vi "Send Email Notification.vi"(5 "Send Email Notification":bool, 7 "Email Notification Cluster (in)":T1, 8 "Error IN":errorcluster, 9 "message":string, 10 "Email Subject":string="[No Subject]", 11 "recipients":string[](array[string])) -> (0 "error out":errorcluster)   [LabVIEW 2012]
uses:
  Controls/Ping address and email notify.ctl
  NewNI_SMTPEmail.lvlib
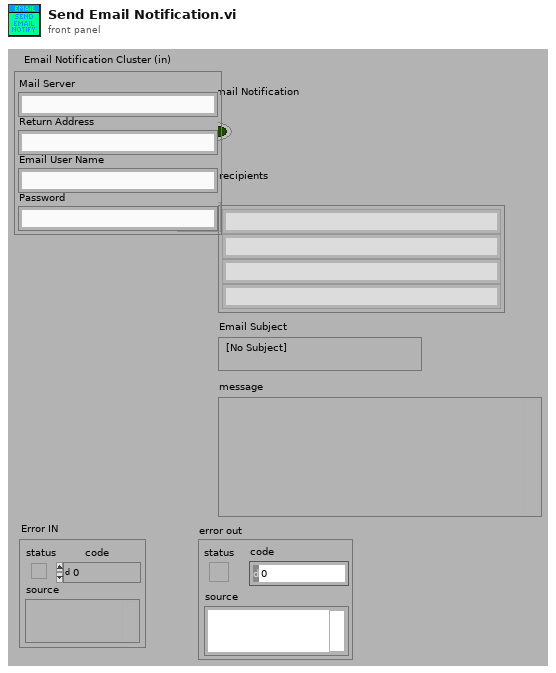
[diagram p1: front panel]
types:
  T1 = typedef "Ping address and email notify.ctl" = cluster{"Mail Server":string, "Return Address":string, "Email User Name":string, "Password":string}
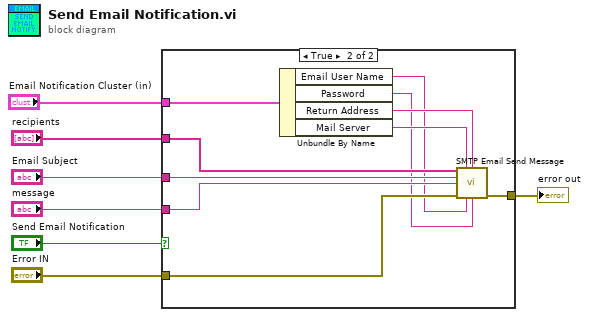
[diagram p0: block diagram]
diagram:
  n1 = case shown="True" "Send Email Notification" {
    tunnel: "recipients" -> [_ w18]
    tunnel: "Email Notification Cluster (in)" -> [_ w17]
    tunnel: [w8 w16] -> w1
    tunnel: "Error IN" -> [w8 w15]
    tunnel: "Email Subject" -> [_ w14]
    tunnel: "message" -> [_ w13]
    frame False {
    }
    frame True {
      n2 = Unbundle By Name(w17) -> ("Email User Name"=w9:string, "Password"=w10:string, "Return Address"=w11:string, "Mail Server"=w12:string)
      n3 = call "SMTP Email Send Message.vi"("recipients"=w18, "mail server"=w12, "return address"=w11, "subject ([No Subject])"=w14, "message"=w13, "error in (no error)"=w15, "username"=w9, "password"=w10) -> ("error out"=w16:errorcluster)  [unwired: 7 out]
    }
  }
  "error out" <- w1
